vi "Initialize Instrument.vi"(8 "error in (no error)":errorcluster, 10 "Reset":bool, 11 "Keithley 2100 in":refnum<class "Keithley 2100.lvclass">) -> (0 "error out":errorcluster, 3 "Keithley 2100 out":refnum<class "Keithley 2100.lvclass">)   [LabVIEW 2020, in "Keithley 2100.lvclass"]
uses:
  Keithley 2100.lvclass
  C:/Sandbox/RF Bench/Source Code/WiSpry Test Framework/Instruments/Instrument.lvclass
  Instrument.lvclass/Instrument.ctl
  Instrument.lvclass
  <instrlib>/Keithley 2100 Series/Keithley 2100 Series.lvlib
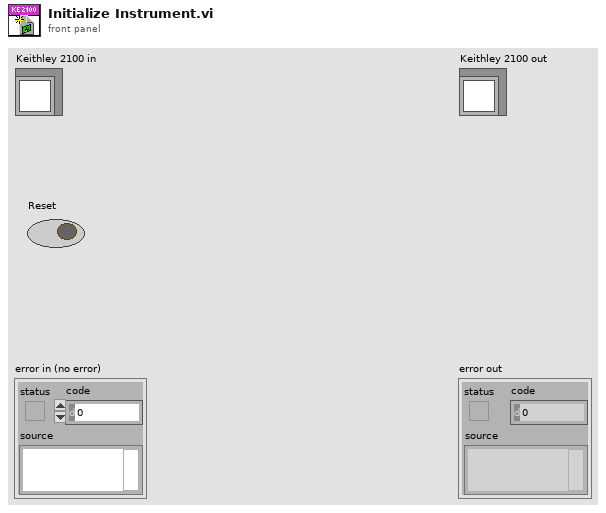
[diagram p1: front panel]
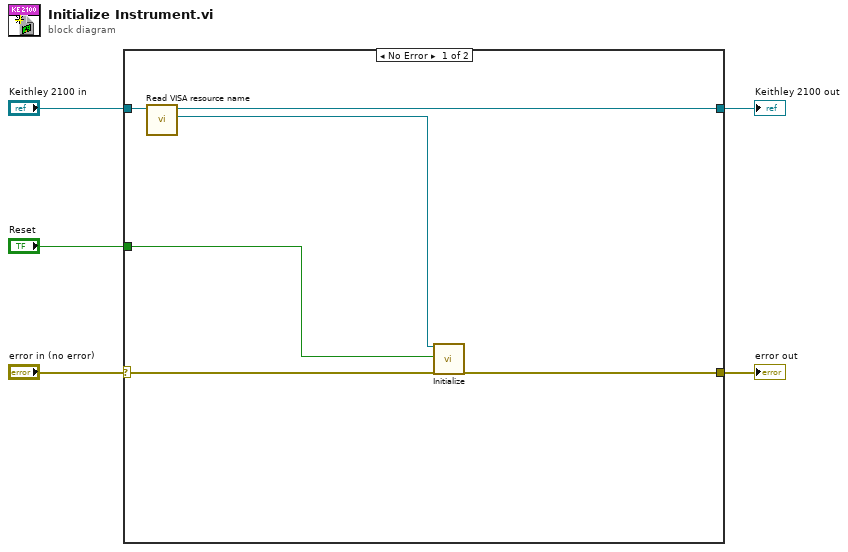
[diagram p0: block diagram]
diagram:
  n1 = case shown="No Error" "error in (no error)" {
    selector: "error in (no error)" -> [w7 w13]
    tunnel: [w8 w13] -> w3
    tunnel: [w10 w12] -> w2
    tunnel: "Keithley 2100 in" -> [w11 w12]
    tunnel: "Reset" -> [w6 _]
    frame No Error {
      n2 = call "Read VISA resource name.vi"("Instrument in"=w11) -> ("VISA resource name"=w9:refnum<visa-resource-name>, "Instrument out"=w10:refnum<class "Keithley 2100.lvclass">)  [unwired: 9 in]
      n3 = call <instrlib>:"Initialize.vi"("VISA resource name"=w9, "Reset? (T: Reset)"=w6, "error in (no error)"=w7) -> ("error out"=w8:errorcluster)  [unwired: 15 in, 1 out]
    }
    frame Error {
    }
  }
  "error out" <- w3
  "Keithley 2100 out" <- w2
